vi "stringArrayToStringWithBrackets.vi"(8 "error in (no error)":errorcluster, 11 "value":string[](array[string])=["uno", "dos"]) -> (0 "error out":errorcluster, 3 "String":string)   [LabVIEW 2018]
doc: "Convert a string array of 1-dimension to a table in string form separated by comma and between brackets."
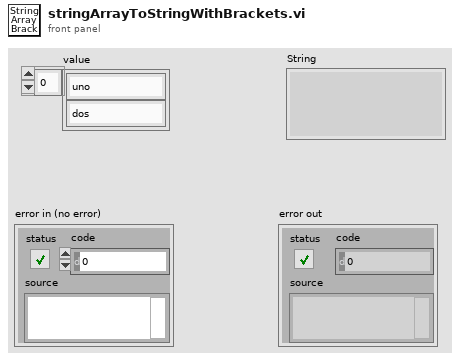
[diagram p1: front panel]
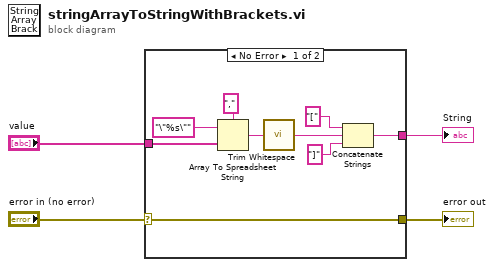
[diagram p0: block diagram]
diagram:
  n1 = case shown="No Error" "error in (no error)" {
    selector: "error in (no error)" -> [w7 w14]
    tunnel: [w13 _] -> w4
    tunnel: [w7 w14] -> w2
    tunnel: "value" -> [w5 _]
    frame No Error {
      n2 = Array To Spreadsheet String(delimiter (Tab)=",", array=w5, 3:"\"%s\"" ("format string")) -> (spreadsheet string=w9:string)
      n3 = call <vilib>:"Trim Whitespace.vi"("string"=w9) -> ("trimmed string"=w12:string)  [unwired: 1 in]
      n4 = Concatenate Strings("[" ("string"), w12, "]" ("string")) -> (w13:string)
    }
    frame Error {
    }
  }
  "String" <- w4
  "error out" <- w2
